vi "plot_selector6.vi"(0 "smooth":u16(ring) items=["origin"=0, "orig&med"=5, "orig-med"=6, "orig&poly"=1, "orig-poly"=3, "polynom"=2, "median"=4], 2 "drawshift":i32, 3 "allinfos":T1(array[cluster]), 4 "legent-plot":T2={"LegendON"=FALSE, "path-name"=FALSE, "aver.\ncolor"=16777215, "width"=0} {"width" min=0 max=5 step=1}, 5 "inp.control":T3(array[cluster]) {"width" min=0 max=5 step=1; "Y-shift" format="%.4f"; "dataname" items=["***", "35#2\\cleaning", "35#4\\cleaning", "35#6\\cleaning", "35#10\\cleaning", "_0034_E-2010_4R235953#1\\Cleaning", "_0034_E-2010_4R235953#2\\Cleaning", "_0034_E-2010_4R235953#3\\Cleaning", "_0034_E-2010_4R235953#4\\Cleaning"]}, 6 "data view":refnum<vi>) -> (1 "data#inp.control#":cluster{"data #":i32[], "inp.control#":i32[]})   [LabVIEW 2014]
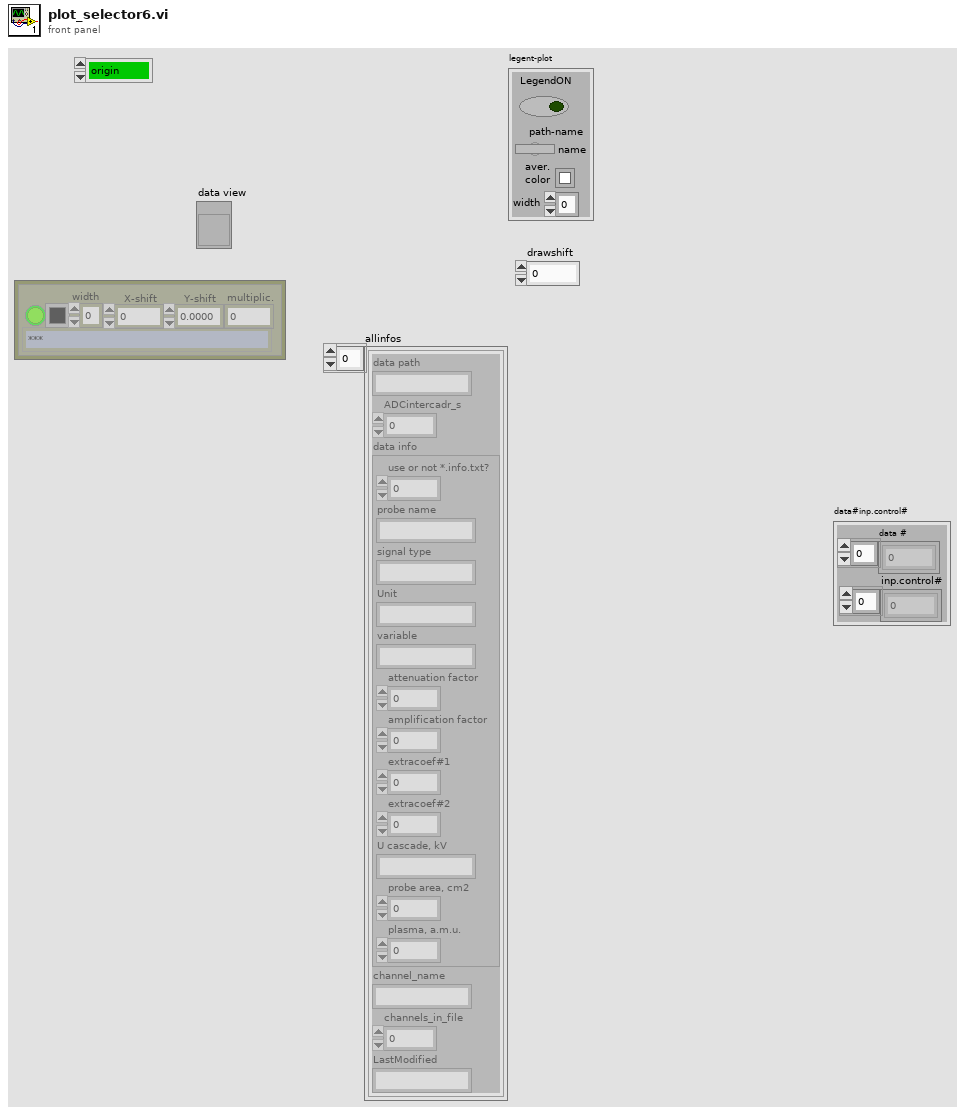
[diagram p1: front panel]
types:
  T1 = cluster{"data path":string, "ADCintercadr_s":dbl, "data info":cluster{"use or not *.info.txt?":i16, "probe name":string, "signal type":string, "Unit":string, "variable":string, "attenuation factor":dbl, "amplification factor":dbl, "extracoef#1":dbl, "extracoef#2":dbl, "U cascade, kV":string, "probe area, cm2":dbl, "plasma, a.m.u.":dbl}, "channel_name":string, "channels_in_file":i32, "LastModified":string}[]
  T2 = cluster{"LegendON":bool, "path-name":bool, "aver.\ncolor":u32, "width":i16}
  T3 = cluster{"dataname":u16, "X-shift":i32, "Y-shift":dbl, "width":i16, "Color":u32, "visible":bool, "multiplic.":dbl}[]
  T4 = cluster{"data path":string, "ADCintercadr_s":dbl, "data info":cluster{"use or not *.info.txt?":i16, "probe name":string, "signal type":string, "Unit":string, "variable":string, "attenuation factor":dbl, "amplification factor":dbl, "extracoef#1":dbl, "extracoef#2":dbl, "U cascade, kV":string, "probe area, cm2":dbl, "plasma, a.m.u.":dbl}, "channel_name":string, "channels_in_file":i32, "LastModified":string}
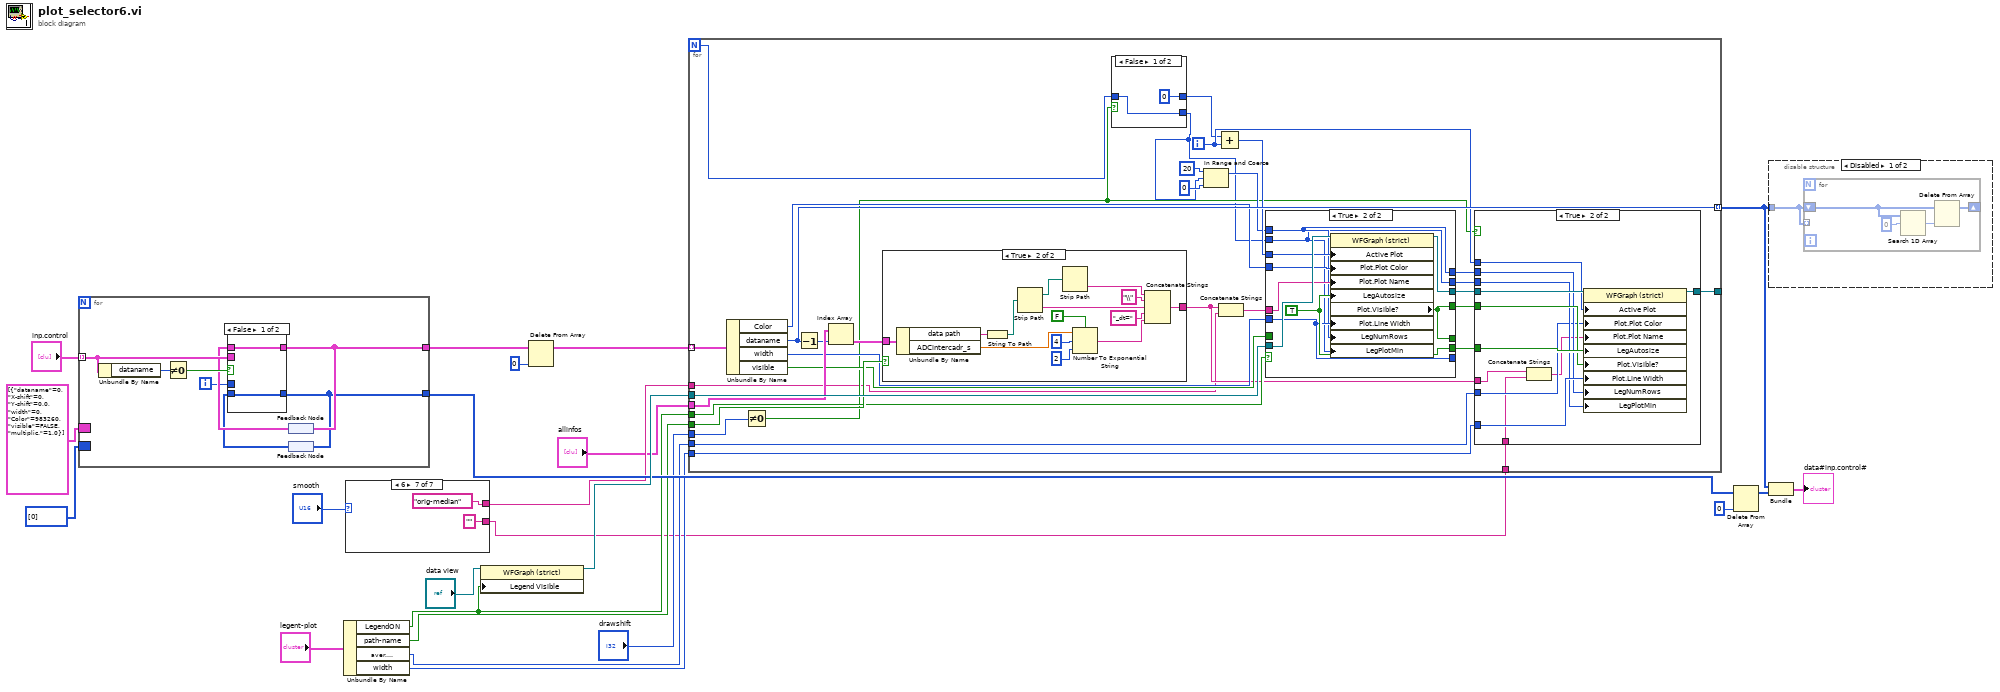
[diagram p0: block diagram]
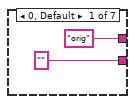
[diagram p2: hidden frame]
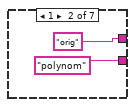
[diagram p3: hidden frame]
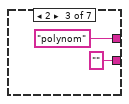
[diagram p4: hidden frame]
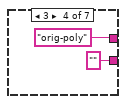
[diagram p5: hidden frame]
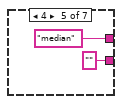
[diagram p6: hidden frame]
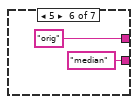
[diagram p7: hidden frame]
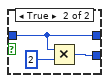
[diagram p8: hidden frame]
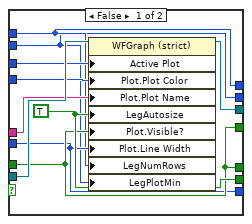
[diagram p10: hidden frame]
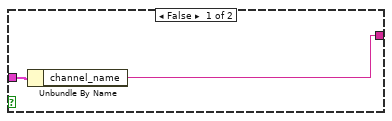
[diagram p11: hidden frame]
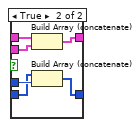
[diagram p13: hidden frame]
diagram:
  n1 = for {
    tunnel: "inp.control" -> [w29] mode=indexing
    tunnel: [w27] -> w18
    border: T3 [{"dataname"=0, "X-shift"=0, "Y-shift"=0.0, "width"=0, "Color"=983260, "visible"=FALSE, "multiplic."=1.0}] ("inp.control") -> [_]
    border: i32[] [0] -> [_]
    tunnel: [w24] -> w15
    i -> [w26]
    n2 = Unbundle By Name(w29) -> ("dataname"=w31:u16)
    n3 = Not Equal To 0?(x=w31) -> (x != 0?=w30:bool)
    n4 = feedback #1() -> (w28:T3)
    n5 = feedback #2() -> (w25:i32[])
    n6 = case shown="False" w30 {
      tunnel: w29 -> [_ w38]
      tunnel: [w33 w37] -> w27
      tunnel: w28 -> [w33 w39]
      tunnel: w26 -> [_ w36]
      tunnel: [w32 w35] -> w24
      tunnel: w25 -> [w32 w34]
      frame False {
      }
      frame True {
        n7 = Build Array (concatenate)(w39, w38) -> (w37:T3)
        n8 = Build Array (concatenate)(w34, w36) -> (w35:i32[])
      }
    }
    n9 = feedback-in #1(w27) -> ()
    n10 = feedback-in #2(w24) -> ()
  }
  n11 = Unbundle By Name("legent-plot") -> ("LegendON"=w8:bool, "path-name"=w7:bool, "aver.\ncolor"=w6:u32, "width"=w5:i16)
  n12 = case shown="6" "smooth" {
    tunnel: ["orig" "orig" "polynom" "orig-poly" "median" "orig" "orig-median"] -> w3
    tunnel: ["" "polynom" "" "" "" "median" ""] -> w2
    frame 0, Default {
    }
    frame 1 {
    }
    frame 2 {
    }
    frame 3 {
    }
    frame 4 {
    }
    frame 5 {
    }
    frame 6 {
    }
  }
  n13 = property class="WFGraph (strict)"(reference="data view", "Legend Visible"=w8) -> (reference out=w19:refnum<vi>)  [unwired: 1 in, 1 out]
  n14 = Delete From Array(array=w18, index=0 ("length")) -> (array with subset deleted=w16:T3)  [unwired: 1 in, 1 out]
  n15 = for {
    N -> [w60]
    tunnel: w19 -> [w86]
    tunnel: w16 -> [w85] mode=indexing
    tunnel: [w83] -> w11 mode=indexing
    tunnel: "allinfos" -> [w84]
    tunnel: w7 -> [w81]
    tunnel: "drawshift" -> [w64]
    tunnel: w8 -> [w72]
    tunnel: w6 -> [w65]
    tunnel: w5 -> [w63]
    tunnel: [w62] -> _
    tunnel: w3 -> [w56]
    tunnel: w2 -> [w55]
    i -> [w70]
    n16 = Unbundle By Name(w85) -> ("Color"=w76:u32, "dataname"=w83:u16, "width"=w75:i16, "visible"=w73:bool)
    n17 = Not Equal To 0?(x=w64) -> (x != 0?=w61:bool)
    n18 = Decrement(x=w83) -> (x-1=w82:u16)
    n19 = Index Array(array=w84, index=w82) -> (element=w80:T4)
    n20 = case shown="True" w81 {
      tunnel: w80 -> [w126 w140]
      tunnel: [w125 w128] -> w57
      frame False {
        n21 = Unbundle By Name(w126) -> ("channel_name"=w125:string)
      }
      frame True {
        n22 = Unbundle By Name(w140) -> ("data path"=w139:string, "ADCintercadr_s"=w132:dbl)
        n23 = String To Path(string=w139) -> (path=w138:path)
        n24 = Strip Path(path=w138) -> (stripped path=w137:path, name=w134:string)
        n25 = Strip Path(path=w137) -> (name=w136:string)  [unwired: 1 out]
        n26 = Number To Exponential String(number=w132, precision (6)=i16 2, 1:FALSE ("use system decimal point (T)"), 3:i16 4 ("width (-)")) -> (E-format string=w129:string)
        n27 = Concatenate Strings(w136, "\\" ("string"), w134, "_dt=" ("string"), w129) -> (w128:string)
      }
    }
    n28 = case shown="False" w61 {
      tunnel: w60 -> [w87 w91]
      tunnel: [0 w91] -> w59
      tunnel: [w87 w89] -> w54
      frame False {
      }
      frame True {
        n29 = Multiply(x=w91, y=2) -> (x*y=w89:i32)
      }
    }
    n30 = In Range and Coerce(upper limit=20, x=w54, lower limit=0) -> (coerced(x)=w74:i32)  [unwired: 1 out]
    n31 = Add(x=w59, y=w70) -> (x+y=w77:i32)
    n32 = Concatenate Strings(w57, w56) -> (w58:string)
    n33 = case shown="True" w72 {
      tunnel: w86 -> [w114 w124]
      tunnel: w77 -> [w113 w123]
      tunnel: w76 -> [w112 w122]
      tunnel: w58 -> [w110 w120]
      tunnel: w75 -> [w107 w117]
      tunnel: w74 -> [w106 w116]
      tunnel: w54 -> [w105 w115]
      tunnel: w73 -> [w108 _]
      tunnel: [w108 w118] -> _
      tunnel: [w111 w121] -> w71
      tunnel: [w109 w119] -> w69
      tunnel: [w108 w118] -> w68
      tunnel: [w107 w117] -> _
      tunnel: [w106 w116] -> w67
      tunnel: [w105 w115] -> w66
      frame False {
        w109 = TRUE ("Legend:Autosize")
        n34 = property on="Property Node" class="WFGraph (strict)"(reference=w114, "Active Plot"=w113, "Plot.Plot Color"=w112, "Plot.Plot Name"=w110, "LegAutosize"=w109, "Plot.Visible?"=w108, "Plot.Line Width"=w107, "LegNumRows"=w106, "LegPlotMin"=w105) -> (reference out=w111:refnum<vi>)  [unwired: 1 in, 1 out]
      }
      frame True {
        w119 = TRUE ("Legend:Autosize")
        n35 = property on="Property Node" class="WFGraph (strict)"(reference=w124, "Active Plot"=w123, "Plot.Plot Color"=w122, "Plot.Plot Name"=w120, "LegAutosize"=w119, "Plot.Line Width"=w117, "LegNumRows"=w116, "LegPlotMin"=w115) -> (reference out=w121:refnum<vi>, "Plot.Visible?"=w118:bool)  [unwired: 1 in, 1 out]
      }
    }
    n36 = case shown="True" w61 {
      tunnel: w71 -> [w92 w104]
      tunnel: w70 -> [_ w103]
      tunnel: w57 -> [_ w95]
      tunnel: w69 -> [_ w102]
      tunnel: w68 -> [_ w101]
      tunnel: w63 -> [_ w100]
      tunnel: w67 -> [_ w99]
      tunnel: w66 -> [_ w98]
      tunnel: w65 -> [_ w97]
      tunnel: [w92 w96] -> w62
      tunnel: w55 -> [_ w93]
      frame False {
      }
      frame True {
        n37 = Concatenate Strings(w95, w93) -> (w94:string)
        n38 = property on="Property Node" class="WFGraph (strict)"(reference=w104, "Active Plot"=w103, "Plot.Plot Color"=w97, "Plot.Plot Name"=w94, "LegAutosize"=w102, "Plot.Visible?"=w101, "Plot.Line Width"=w100, "LegNumRows"=w99, "LegPlotMin"=w98) -> (reference out=w96:refnum<vi>)  [unwired: 1 in, 1 out]
      }
    }
  }
  n39 = Delete From Array(array=w15, index=0) -> (array with subset deleted=w12:i32[])  [unwired: 1 in, 1 out]
  n40 = disable-structure shown="Disabled" {
    disable-tunnel: w11 -> [w141 _]
    frame Disabled {
      n41 = for {
        tunnel: w141 -> [_] mode=indexing
        shift-right: [w143] -> _
        shift-left: w141 -> [w142]
        n42 = Search 1D Array(1D array=w142, element=u16 0) -> (index of element=w144:i32)  [unwired: 1 in]
        n43 = Delete From Array(array=w142, index=w144) -> (array with subset deleted=w143:u16[])  [unwired: 1 in, 1 out]
      }
    }
    frame Enabled {
    }
  }
  n44 = Bundle(w11, w12) -> (→"data#inp.control#":cluster{u16[], i32[]})  [unwired: 1 in]
